vi "Set Signal Results Names.vi"(8 "error in (no error)":errorcluster, 9 "Meas Step Ref":refnum<k7>, 10 "Fetch Step Ref":refnum<k7>, 11 "NF in":refnum<class "NF.lvclass">) -> (0 "error out":errorcluster, 1 "Meas Step Ref":refnum<k7>, 2 "Fetch Step Ref":refnum<k7>, 3 "NF out":refnum<class "NF.lvclass">)   [LabVIEW 2018, in "NF.lvlib" / "NF.lvclass"]
uses:
  NF.lvclass
  NF.lvclass/NF.ctl
  Read Signal Name.vi
  Plugins/TestStand API Tools (TSAT).lvlibp/Step Actions/TSAT Step Actions.lvlib
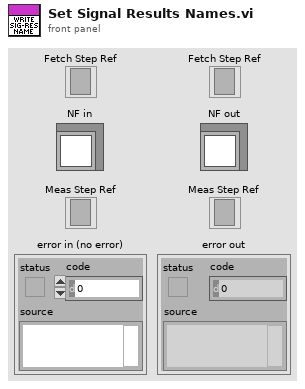
[diagram p1: front panel]
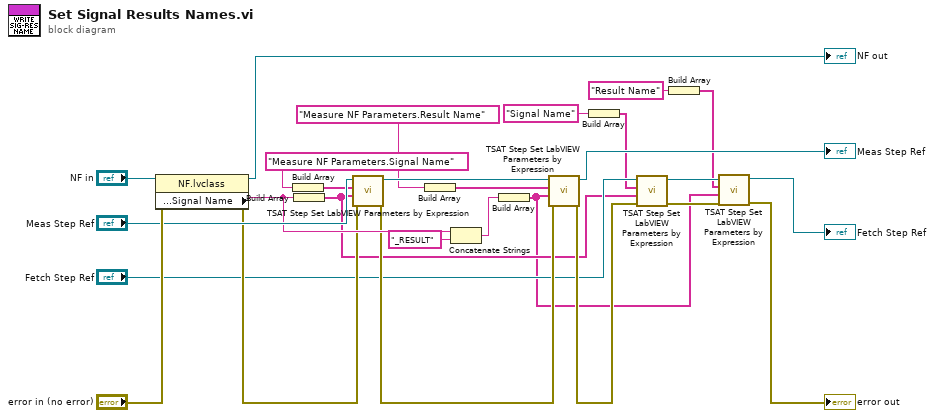
[diagram p0: block diagram]
diagram:
  n1 = property class="NF.lvclass"(reference="NF in", error in="error in (no error)") -> (reference out=→"NF out":refnum<class "NF.lvclass">, error out=w19:errorcluster, "Private Methods:Signal Name"=w22:string)
  n2 = Build Array("Measure NF Parameters.Signal Name" ("LabVIEW Parameter to Set")) -> (w8:string[])
  n3 = Build Array(w22) -> (w12:string[])
  n4 = call "TSAT Step Set LabVIEW Parameters by Expression.vi"("Error In"=w19, "Value Expressions"=w12, "Parameters to Set"=w8, "Step In"="Meas Step Ref") -> ("Error Out"=w18:errorcluster, "Step Out"=w25:refnum<k7>)  [unwired: 6 in]
  n5 = Build Array("Measure NF Parameters.Result Name" ("LabVIEW Parameter to Set")) -> (w6:string[])
  n6 = Concatenate Strings(w22, "_RESULT" ("string")) -> (w20:string)
  n7 = Build Array(w20) -> (w11:string[])
  n8 = call "TSAT Step Set LabVIEW Parameters by Expression.vi"("Error In"=w18, "Value Expressions"=w11, "Parameters to Set"=w6, "Step In"=w25) -> ("Error Out"=w16:errorcluster, "Step Out"=→"Meas Step Ref":refnum<k7>)  [unwired: 6 in]
  n9 = Build Array("Signal Name" ("LabVIEW Parameter to Set")) -> (w4:string[])
  n10 = call "TSAT Step Set LabVIEW Parameters by Expression.vi"("Error In"=w16, "Value Expressions"=w12, "Parameters to Set"=w4, "Step In"="Fetch Step Ref") -> ("Error Out"=w17:errorcluster, "Step Out"=w13:refnum<k7>)  [unwired: 6 in]
  n11 = Build Array("Result Name" ("LabVIEW Parameter to Set")) -> (w2:string[])
  n12 = call "TSAT Step Set LabVIEW Parameters by Expression.vi"("Error In"=w17, "Value Expressions"=w11, "Parameters to Set"=w2, "Step In"=w13) -> ("Error Out"=→"error out":errorcluster, "Step Out"=→"Fetch Step Ref":refnum<k7>)  [unwired: 6 in]
